vi "Point getValues.vi"(0 "point2D":T1 {"y" format="%.2f"; "x" format="%.2f"}) -> (14 "x":dbl format="%.2f", 15 "y":dbl format="%.2f", 16 "valid":bool)   [LabVIEW 2020]
doc: "Get Values"
uses:
  <resource>/Framework/Providers/Open_GDS/UML/General/Point/Point Point2D.ctl
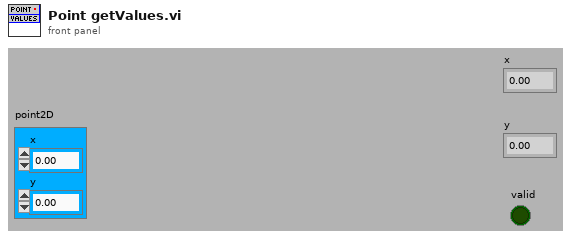
[diagram p1: front panel]
types:
  T1 = typedef "Point Point2D.ctl" = cluster{"x":dbl, "y":dbl}
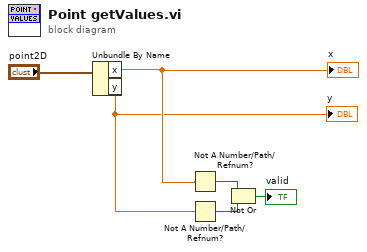
[diagram p0: block diagram]
diagram:
  n1 = Unbundle By Name("point2D") -> ("x"=w5:dbl, "y"=w4:dbl)
  "x" <- w5
  "y" <- w4
  n2 = Not A Number/Path/Refnum?(number/path/refnum=w5) -> (NaN/Path/Refnum?=w3:bool)
  n3 = Not A Number/Path/Refnum?(number/path/refnum=w4) -> (NaN/Path/Refnum?=w2:bool)
  n4 = Not Or(1:w2, 2:w3) -> (0:→"valid":bool)
